vi "Breadth-first search day 16 fast no cache.vi"(9 "distance graph":T2(array[cluster]), 10 "Flow, bitfield":cluster{"flow":i32, "bitfield":u32}[](array[cluster]), 11 "input \n[index, bitfield, time left]":T1) -> (2 "most pressure":i32)   [LabVIEW 2023]
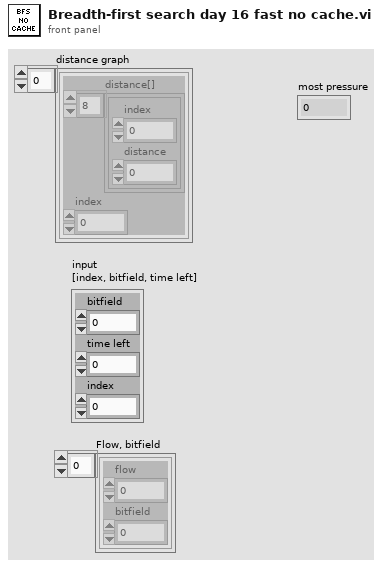
[diagram p1: front panel]
types:
  T1 = cluster{"bitfield":u32, "time left":i32, "index":i32}
  T2 = cluster{"distance[]":cluster{"index":i32, "distance":i32}[], "index":i32}[]
  T3 = cluster{"distance[]":cluster{"index":i32, "distance":i32}[], "index":i32}
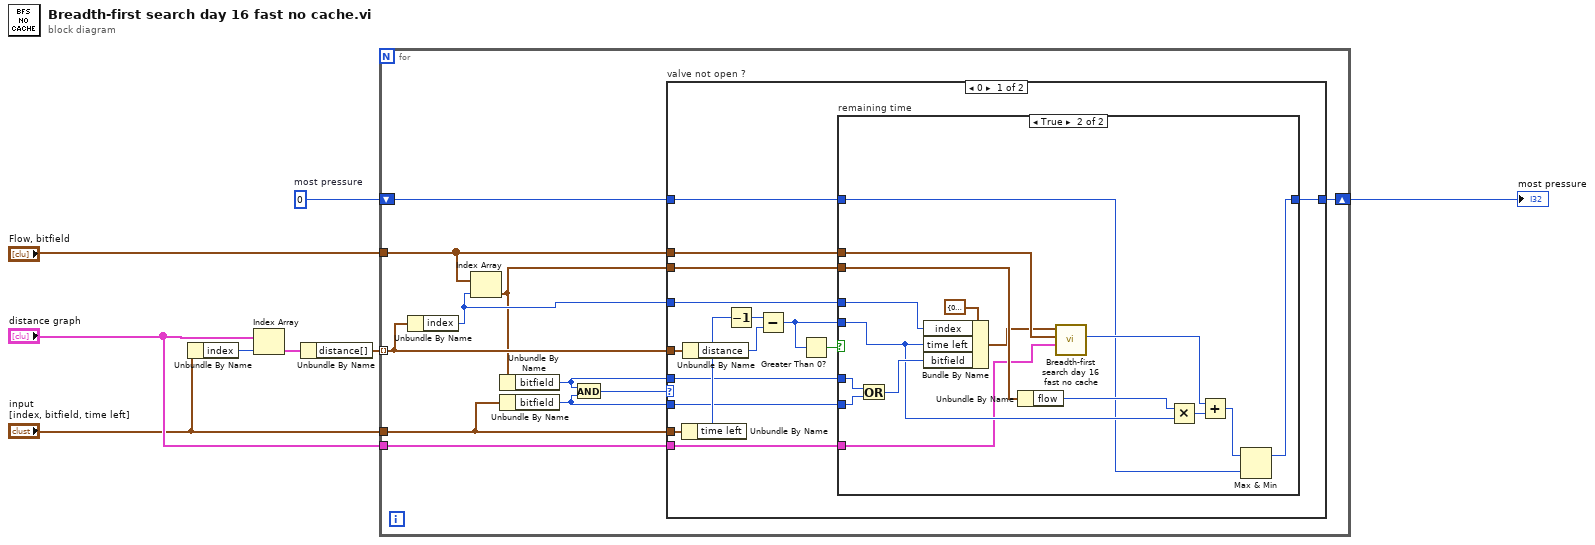
[diagram p0: block diagram]
diagram:
  w4 = 0  # most pressure
  n1 = Unbundle By Name("input \n[index, bitfield, time left]") -> ("index"=w2:i32)
  n2 = Index Array(array="distance graph", index=w2) -> (element=w3:T3)
  n3 = Unbundle By Name(w3) -> ("distance[]"=w1:cluster{"index":i32, "distance":i32}[])
  n4 = for {
    shift-right: [w19] -> w8
    shift-left: w4 -> [w18]
    tunnel: "input \n[index, bitfield, time left]" -> [w15]
    tunnel: w1 -> [w16] mode=indexing
    tunnel: "Flow, bitfield" -> [w10]
    tunnel: "distance graph" -> [w9]
    n5 = Unbundle By Name(w16) -> ("index"=w12:i32)
    n6 = Index Array(array=w10, index=w12) -> (element=w11:cluster{"flow":i32, "bitfield":u32})
    n7 = Unbundle By Name(w11) -> ("bitfield"=w13:u32)
    n8 = Unbundle By Name(w15) -> ("bitfield"=w14:u32)
    n9 = And(x=w13, y=w14) -> (x .and. y?=w17:u32)
    n10 = case "valve not open ?" shown="0" w17 {
      tunnel: [w34 w52] -> w19
      tunnel: w18 -> [w33 w52]
      tunnel: w16 -> [w30 _]
      tunnel: w15 -> [w29 _]
      tunnel: w14 -> [w25 _]
      tunnel: w13 -> [w24 _]
      tunnel: w12 -> [w23 _]
      tunnel: w11 -> [w22 _]
      tunnel: w10 -> [w21 _]
      tunnel: w9 -> [w20 _]
      frame 0 {
        n11 = Unbundle By Name(w29) -> ("time left"=w28:i32)
        n12 = Unbundle By Name(w30) -> ("distance"=w32:i32)
        n13 = Decrement(x=w28) -> (x-1=w31:i32)
        n14 = Subtract(x=w31, y=w32) -> (x-y=w26:i32)
        n15 = Greater Than 0?(x=w26) -> (x > 0?=w27:bool)
        n16 = case "remaining time" shown="True" w27 {
          tunnel: [w35 w36] -> w34
          tunnel: w33 -> [w35 w39]
          tunnel: w26 -> [_ w40]
          tunnel: w25 -> [_ w50]
          tunnel: w24 -> [_ w49]
          tunnel: w23 -> [_ w47]
          tunnel: w22 -> [_ w43]
          tunnel: w21 -> [_ w42]
          tunnel: w20 -> [_ w37]
          frame False {
          }
          frame True {
            n17 = Or(x=w49, y=w50) -> (x .or. y?=w48:u32)
            n18 = Bundle By Name(cluster=T1 {"bitfield"=0, "time left"=0, "index"=0}, "index"=w47, "time left"=w40, "bitfield"=w48) -> (w38:T1)
            n19 = Unbundle By Name(w43) -> ("flow"=w46:i32)
            n20 = call "Breadth-first search day 16 fast no cache.vi"("distance graph"=w37, "Flow, bitfield"=w42, "input \n[index, bitfield, time left]"=w38) -> ("most pressure"=w41:i32)  [unwired: 8 in]
            n21 = Multiply(x=w46, y=w40) -> (x*y=w44:i32)
            n22 = Add(x=w41, y=w44) -> (x+y=w45:i32)
            n23 = Max & Min(x=w45, y=w39) -> (max(x,y)=w36:i32)  [unwired: 1 out]
          }
        }
      }
      frame 1, Default {
      }
    }
  }
  "most pressure" <- w8
